vi "Inventory-UpdateSuccess.vi"(0 "Raw Data From DB Actor":string[][](array[string]), 1 "Column#":i32, 2 "Data":string, 7 "error in":errorcluster) -> (4 "Update Transaction Complete":bool, 8 "error out":errorcluster)   [LabVIEW 2013, in "ERP-Inventory.lvclass"]
uses:
  ERP-Inventory.lvclass
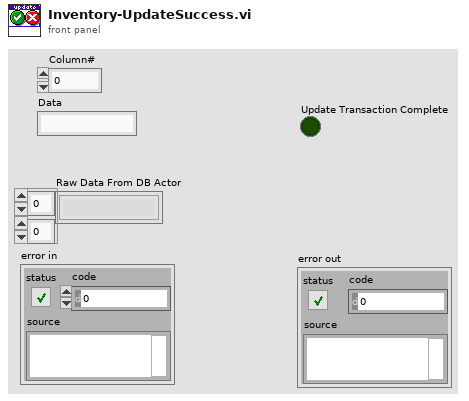
[diagram p1: front panel]
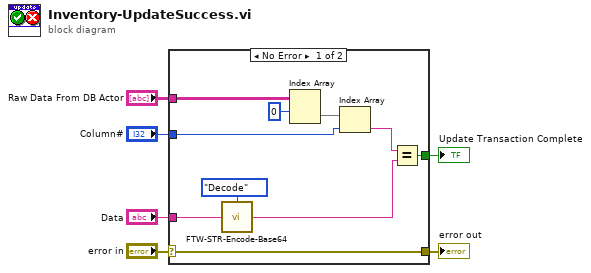
[diagram p0: block diagram]
diagram:
  n1 = case shown="No Error" "error in" {
    selector: "error in" -> [w7 w17]
    tunnel: "Column#" -> [w11 _]
    tunnel: "Raw Data From DB Actor" -> [w10 _]
    tunnel: "Data" -> [w9 _]
    tunnel: [w8 _] -> w2
    tunnel: [w7 w17] -> w1
    frame No Error {
      n2 = call "FTW-STR-Encode-Base64.vi"("Input"=w9, "Direction"=enum16{"Encode", "Decode"}."Decode") -> ("Output"=w12:string)
      n3 = Index Array(array=w10, index (row)=0) -> (element=w14:string[])  [unwired: 1 in]
      n4 = Index Array(array=w14, index=w11) -> (element=w15:string)
      n5 = Equal?(x=w15, y=w12) -> (x = y?=w8:bool)
    }
    frame Error {
    }
  }
  "Update Transaction Complete" <- w2
  "error out" <- w1
